vi "07_jednoduche_prevzorkovani_signalu.vi"() -> ()   [LabVIEW 2019]
uses:
  <vilib>/Analysis/3filter.llb/Filter Passband Type.ctl
  <vilib>/measure/maresamp.llb/Resample Waveform (single shot).vi
  <vilib>/Analysis/3filter.llb/Butterworth Filter (DBL).vi
  <vilib>/measure/NI_MABase.lvlib
  <vilib>/measure/NI_MAPro.lvlib
  <vilib>/Analysis/NI_AALBase.lvlib
panel:
  out "Zaokrouhlena nedokonala Fvz":dbl=500.0
  in  "Nova vzorkovaci frekvence":dbl=500.0 format="%0.2p"
  out "Waveform Graph":waveform(dbl)[](graph)=[{"t0"=timestamp(0 s since 1904-01-01), "dt"=0.0002, "Y"=array[1000 elements]}, {"t0"=timestamp(0 s since 1904-01-01), "dt"=0.002, "Y"=[-0.817270653747393, -0.01726846362672692, 0.7827305238760827, 1.5827309703334245, 2.382730780356192, 3.182730858895974, 3.9827308272220576, 4.782730839712263, 5.582730834890395, 6.382730836713253, 7.182730836038887, 7.982730836282638, 8.782730836196816, 9.576610354943858, 9.711343105810277, 8.786673645632634, 8.027895585225778, 7.21380667742924, 6.418307707533951, 5.6169903584189615, 4.817328114895193, 4.017265437945788, 3.21726331272766, 2.4172741560231366, 1.6172662339646622, 0.8172706537473948, 0.017268463626728722, -0.7827305238760837, -1.5827309703334247, -2.3827307803561917, -3.1827308588959737, -3.982730827222058, -4.782730839712261, -5.582730834890395, -6.3827308367132485, -7.1827308360388855, -7.982730836282631, -8.782730836196817, -9.576610354943849, -9.711343105810272, -8.78667364563264, -8.02789558522577, -7.213806677429243, -6.418307707533951, -5.6169903584189615, -4.817328114895196, -4.017265437945795, -3.2172633127276593, -2.4172741560231357, -1.6172662339646573, -0.8172706537473956, -0.017268463626726446, 0.7827305238760836, 1.5827309703334247, 2.3827307803561917, 3.182730858895969, 3.982730827222059, 4.782730839712262, 5.582730834890393, 6.382730836713259, 7.182730836038892, 7.982730836282634, 8.782730836196816, 9.576610354943844, 9.71134310581028, 8.786673645632643, 8.027895585225773, 7.213806677429243, 6.418307707533943, 5.616990358418961, 4.817328114895193, 4.017265437945797, 3.217263312727658, 2.417274156023135, 1.6172662339646593, 0.8172706537473946, 0.01726846362672707, -0.7827305238760847, -1.582730970333426, -2.3827307803561943, -3.182730858895974, -3.9827308272220634, -4.782730839712262, -5.582730834890398, -6.382730836713253, -7.18273083603889, -7.98273083628263, -8.782730836196823, -9.57661035494385, -9.711343105810275, -8.786673645632638, -8.027895585225775, -7.213806677429227, -6.418307707533945, -5.6169903584189536, -4.817328114895201, -4.017265437945799, -3.2172633127276615, -2.4172741560231343, -1.6172662339646569]}, {"t0"=timestamp(0 s since 1904-01-01), "dt"=0.002, "Y"=[0.0, 0.8, 1.6, 2.4000000000000004, 3.2, 4.0, 4.800000000000001, 5.6000000000000005, 6.4, 7.199999999999999, 8.0, 8.8, 9.600000000000001, 9.6, 8.799999999999999, 8.0, 7.199999999999999, 6.399999999999999, 5.6000000000000005, 4.799999999999997, 3.999999999999999, 3.1999999999999984, 2.3999999999999977, 1.5999999999999992, 0.7999999999999985, 0.0, -0.8000000000000007, -1.6000000000000014, -2.400000000000002, -3.200000000000003, -3.999999999999999, -4.800000000000004, -5.6000000000000005, -6.400000000000001, -7.200000000000002, -8.000000000000004, -8.799999999999999, -9.6, -9.599999999999994, -8.799999999999999, -7.999999999999998, -7.200000000000002, -6.399999999999997, -5.599999999999996, -4.799999999999995, -3.999999999999999, -3.1999999999999984, -2.3999999999999932, -1.599999999999997, -0.7999999999999963, 0.0, 0.7999999999999987, 1.6000000000000039, 2.4000000000000026, 3.200000000000001, 4.0, 4.799999999999999, 5.600000000000004, 6.400000000000002, 7.200000000000002, 8.0, 8.799999999999999, 9.600000000000005, 9.599999999999998, 8.799999999999999, 8.0, 7.199999999999999, 6.399999999999995, 5.599999999999996, 4.799999999999997, 3.999999999999999, 3.2000000000000006, 2.400000000000002, 1.599999999999997, 0.8000000000000052, 0.0, -0.8000000000000052, -1.599999999999997, -2.400000000000002, -3.2000000000000073, -3.999999999999999, -4.800000000000004, -5.6000000000000005, -6.400000000000006, -7.200000000000011, -8.000000000000004, -8.800000000000008, -9.6, -9.599999999999994, -8.79999999999999, -7.999999999999998, -7.199999999999993, -6.400000000000001, -5.599999999999996, -4.799999999999991, -3.999999999999999, -3.199999999999994, -2.400000000000002, -1.599999999999997, -0.7999999999999918]}]
  in  "Amplituda sumu":dbl format="%.2p"
  in  "Info o vzorkovani":T1={"Vzorkovaci frekvence"=5000.0, "Pocet vzorku v okne"=1000.0} {"Vzorkovaci frekvence" format="%.2p"}
  in  "Faze":dbl format="%.2p"
  in  "Amplituda":dbl=10.0 format="%0.2p"
  in  "Frekvence":dbl=10.0 format="%0.2p"
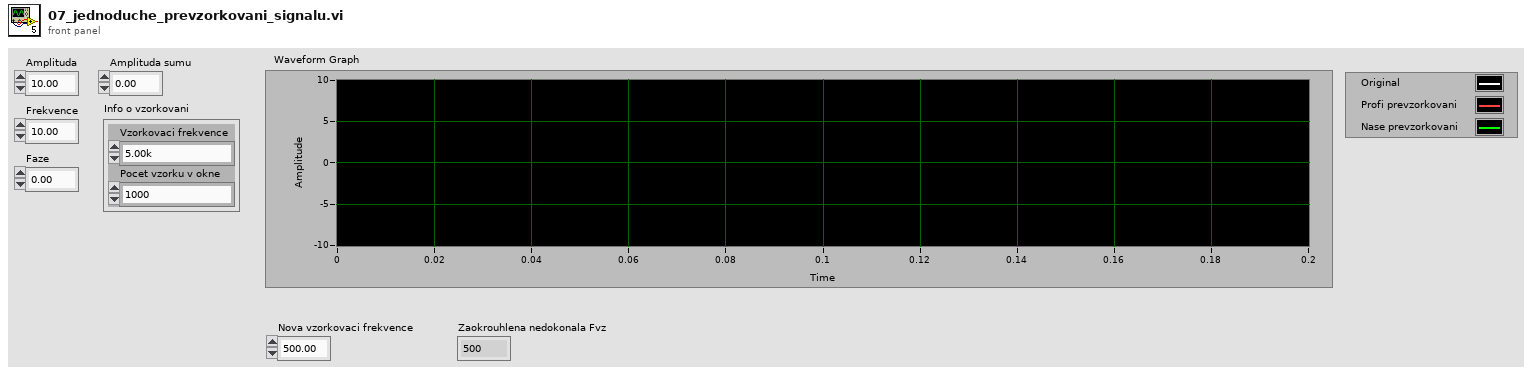
[diagram p1: front panel]
types:
  T1 = cluster{"Vzorkovaci frekvence":dbl, "Pocet vzorku v okne":dbl}
  T2 = typedef "NI_AALBase.lvlib/Filter Passband Type.ctl" = enum32{"Lowpass", "Highpass", "Bandpass", "Bandstop"}
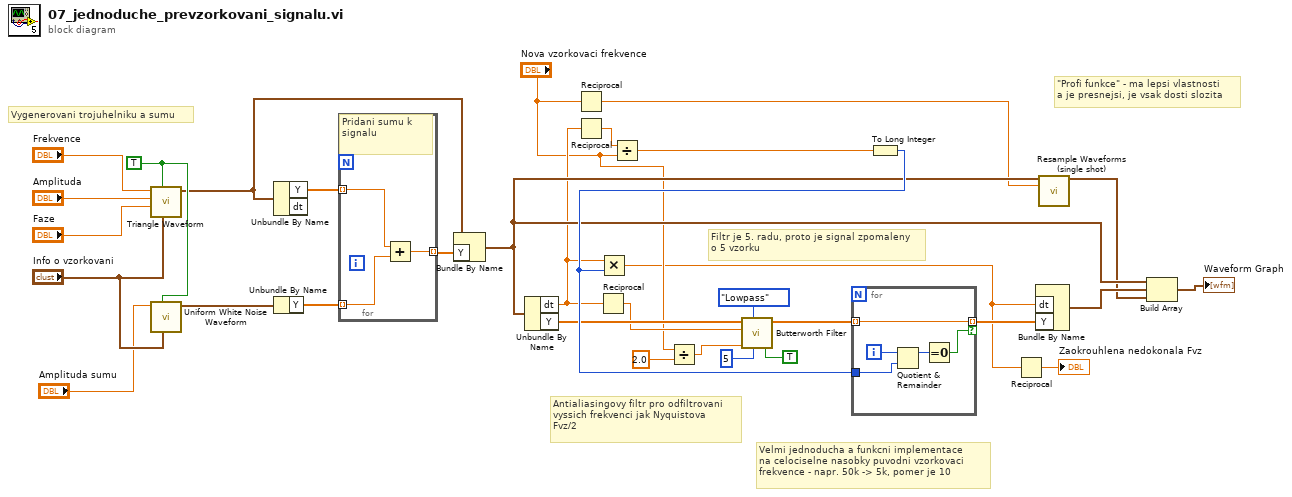
[diagram p0: block diagram]
diagram:
  w27 = TRUE ("reset signal")
  # "Antialiasingovy filtr pro odfiltrovani\nvyssich frekvenci jak Nyquistova\nFvz/2"
  # "Filtr je 5. radu, proto je signal zpomaleny\no 5 vzorku"
  # "Velmi jednoducha a funkcni implementace\nna celociselne nasobky puvodni vzorkovaci \nfrekvence - napr. 50k -> 5k, pomer je 10"
  # "\"Profi funkce\" - ma lepsi vlastnosti\na je presnejsi, je vsak dosti slozita"
  # "Vygenerovani trojuhelniku a sumu"
  n1 = call <vilib>:"Triangle Waveform.vi"("sampling info"="Info o vzorkovani", "reset signal"=w27, "phase"="Faze", "amplitude"="Amplituda", "frequency"="Frekvence") -> ("signal out"=w23:waveform(dbl))  [unwired: 5 in, 1 out]
  n2 = call <vilib>:"Uniform White Noise Waveform.vi"("sampling info"="Info o vzorkovani", "reset signal"=w27, "amplitude"="Amplituda sumu") -> ("signal out"=w26:waveform(dbl))  [unwired: 7 in, 1 out]
  n3 = Unbundle By Name(w23) -> ("Y"=w25:dbl[])  [unwired: 1 out]
  n4 = Unbundle By Name(w26) -> ("Y"=w24:dbl[])
  n5 = for {
    tunnel: w25 -> [w34] mode=indexing
    tunnel: w24 -> [w35] mode=indexing
    tunnel: [w33] -> w22 mode=indexing
    # "Pridani sumu k signalu"
    n6 = Add(x=w34, y=w35) -> (x+y=w33:dbl)
  }
  n7 = Bundle By Name(cluster=w23, "Y"=w22) -> (w16:waveform(dbl))
  n8 = Unbundle By Name(w16) -> ("dt"=w11:dbl, "Y"=w12:dbl[])
  n9 = Reciprocal(x="Nova vzorkovaci frekvence") -> (1/x=w13:dbl)
  n10 = Reciprocal(x=w11) -> (1/x=w14:dbl)
  n11 = Reciprocal(x=w11) -> (1/x=w10:dbl)
  n12 = Divide(x=w14, y="Nova vzorkovaci frekvence") -> (x/y=w18:dbl)
  n13 = Divide(x="Nova vzorkovaci frekvence", y=2.0) -> (x/y=w5:dbl)
  n14 = call-poly <vilib>:"Butterworth Filter.vi"("init/cont (init:F)"=TRUE, "order"=5, "filter type"=Filter_Passband_Type."Lowpass", "low cutoff freq: fl"=w5, "sampling freq: fs"=w10, "X"=w12) -> ("Filtered X"=w8:dbl[])  [unwired: 2 in, 1 out]
  n15 = To Long Integer(number=w18) -> (32bit integer=w17:i32)
  n16 = Multiply(x=w11, y=w17) -> (x*y=w2:dbl)
  n17 = for {
    tunnel: w8 -> [w38] mode=indexing
    tunnel: [w38] -> w21 mode=indexing if=w37
    tunnel: w17 -> [w36]
    i -> [w40]
    n18 = Quotient & Remainder(x=w40, y=w36) -> (x-y*floor(x/y)=w39:i32)  [unwired: 1 out]
    n19 = Equal To 0?(x=w39) -> (x = 0?=w37:bool)
  }
  n20 = Reciprocal(x=w2) -> (1/x=→"Zaokrouhlena nedokonala Fvz":dbl)
  n21 = Bundle By Name("dt"=w2, "Y"=w21) -> (w20:waveform(dbl))  [unwired: 1 in]
  n22 = call-poly <vilib>:"Resample Waveforms (single shot).vi"("waveform in"=w16, "dt"=w13) -> ("resampled waveform out"=w15:waveform(dbl))  [unwired: 10 in, 3 out]
  n23 = Build Array(w16, w20, w15) -> (→"Waveform Graph":waveform(dbl)[])
